vi "PMLambda-Conct Rev A.vi"(0 "Case0:NewFWNone":bool, 1 "Case1:NewFWRed":bool, 2 "Case2:NewFW780":bool, 3 "Case3:NewFW850":bool, 4 "Case4:OldFWRed\nElse5:FW error":bool, 5 "error in":errorcluster, 6 "Supply Cnt":i32=1 min=1 max=5 step=1, 7 "N Systems":i32=1 min=1 max=8 step=1, 8 "COM Ref In":refnum<vi>, 10 "Msg Ref In":refnum<vi>, 11 "Loop Index":i32) -> (14 "Re-conf Lambda?":bool, 15 "Lambda, nm":i32, 19 "error out":errorcluster)   [LabVIEW 2017]
panel:
  # "Inputs"
  # "Outputs"
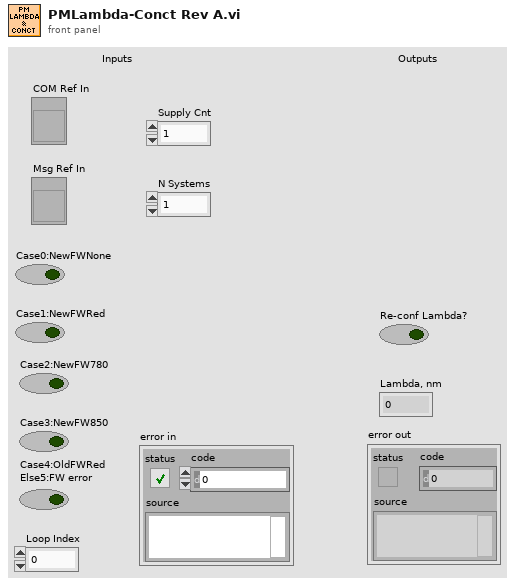
[diagram p1: front panel]
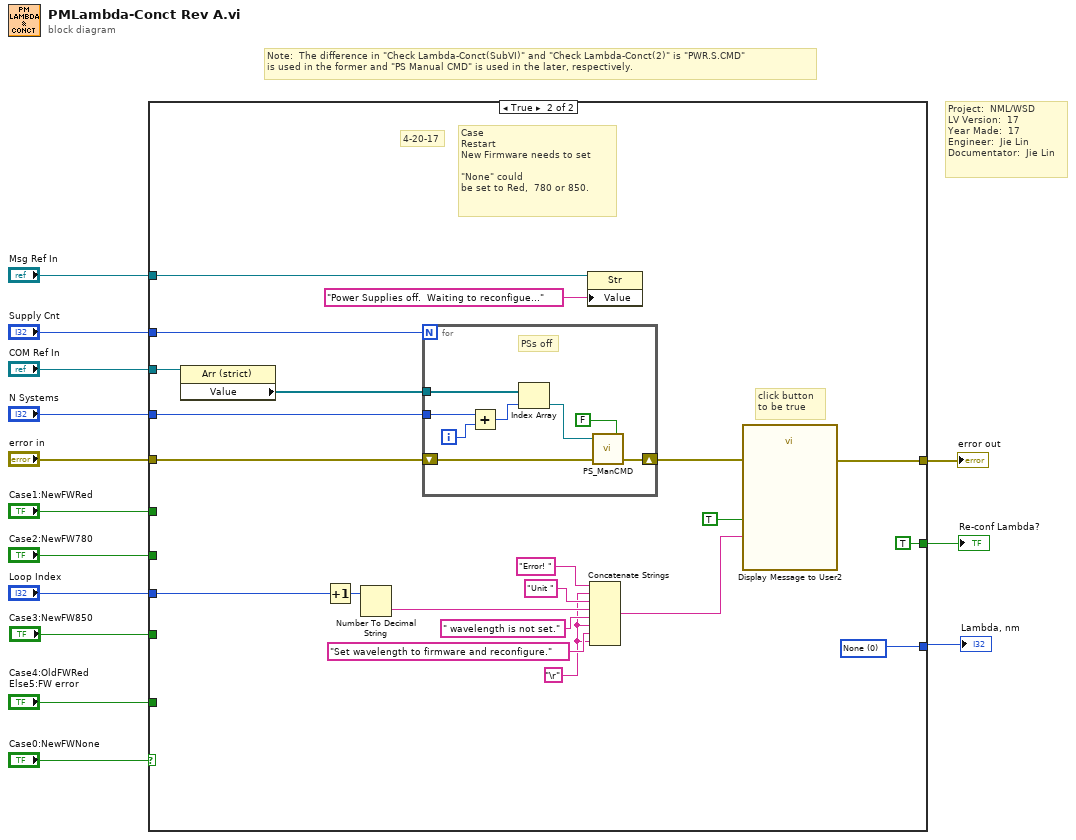
[diagram p0: block diagram]
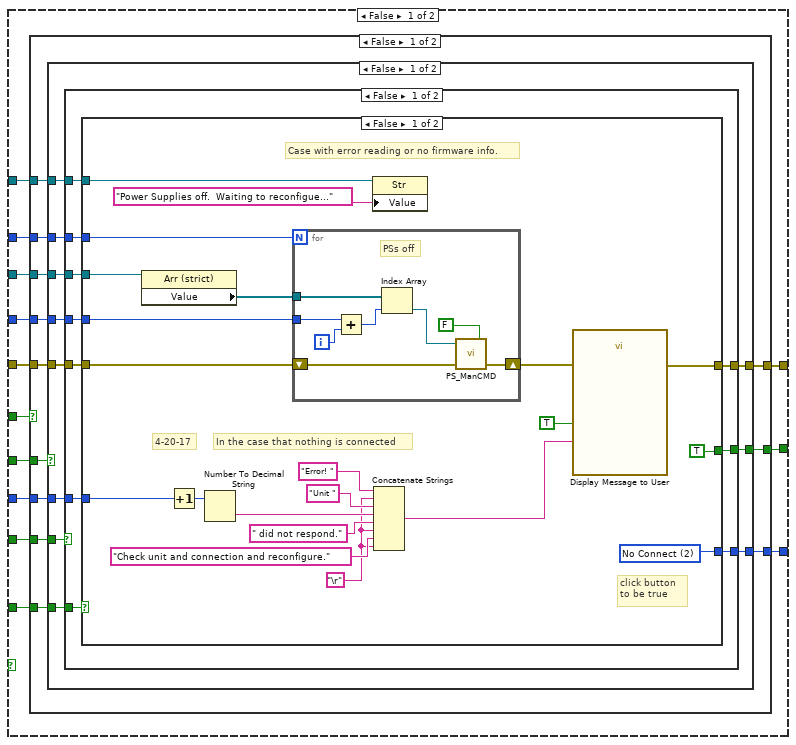
[diagram p2: hidden frame]
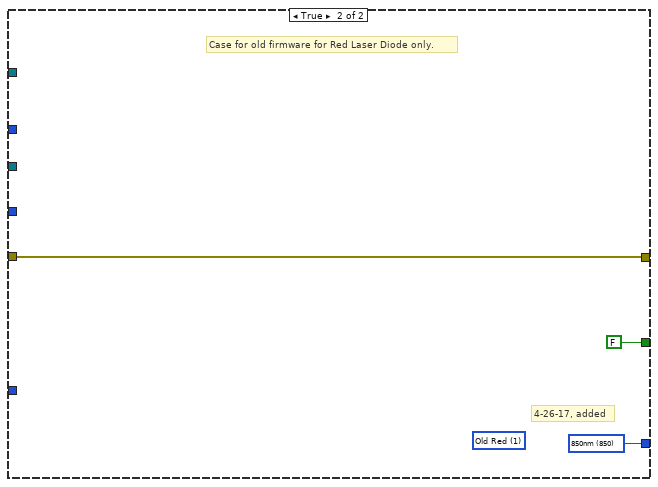
[diagram p3: hidden frame]
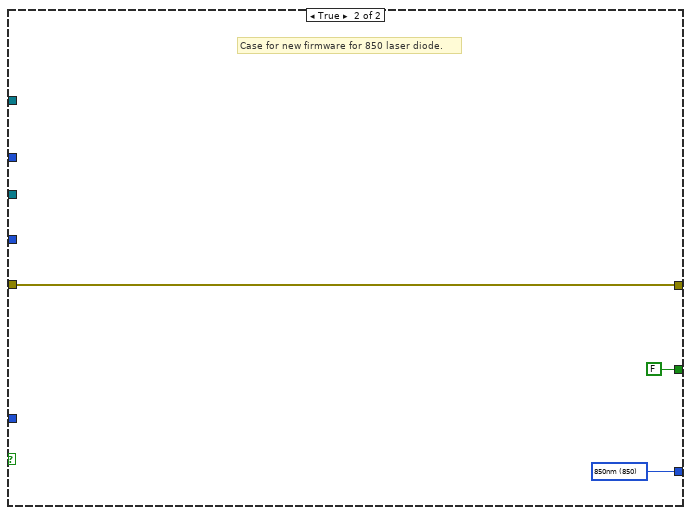
[diagram p4: hidden frame]
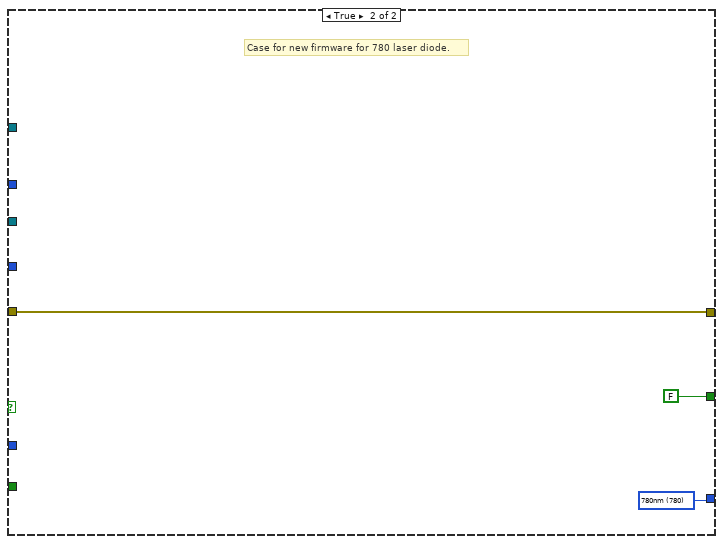
[diagram p5: hidden frame]
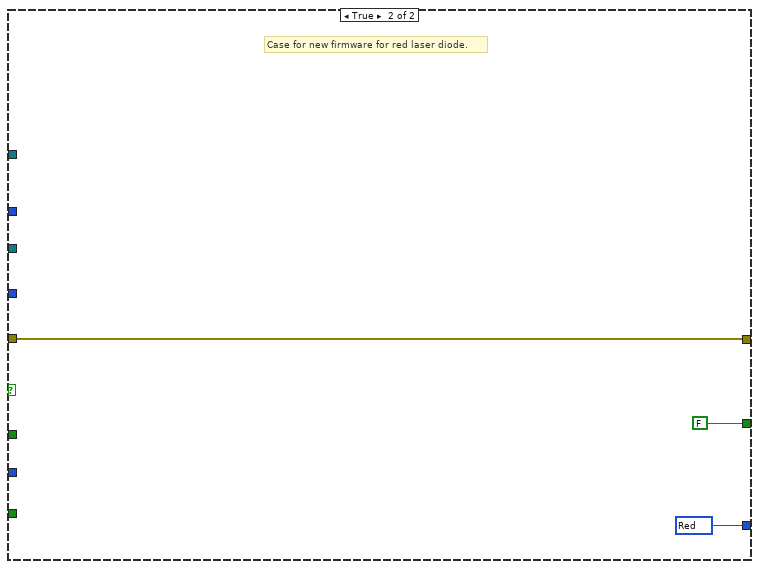
[diagram p6: hidden frame]
diagram:
  # "Project:  NML/WSD \nLV Version:  17\nYear Made:  17\nEngineer:  Jie Lin\nDocumentator:  Jie Lin"
  # "Note:  The difference in \"Check Lambda-Conct(SubVI)\" and \"Check Lambda-Conct(2)\" is \"PWR.S.CMD\" \nis used in the former and \"PS Manual CMD\" is used in the later, respectively."
  n1 = case shown="True" "Case0:NewFWNone" {
    tunnel: [w26 w122] -> w7
    tunnel: "Case1:NewFWRed" -> [w27 _]
    tunnel: "Case2:NewFW780" -> [w25 _]
    tunnel: "Case3:NewFW850" -> [w24 _]
    tunnel: "Case4:OldFWRed\nElse5:FW error" -> [w23 _]
    tunnel: "Loop Index" -> [w17 w113]
    tunnel: [w22 TRUE ("Restart Test")] -> w14
    tunnel: "COM Ref In" -> [w21 w107]
    tunnel: "Msg Ref In" -> [w20 w106]
    tunnel: "error in" -> [w18 w105]
    tunnel: [w19 w104] -> w3
    tunnel: "Supply Cnt" -> [w16 w103]
    tunnel: "N Systems" -> [w15 w102]
    frame False {
      n2 = case shown="False" w27 {
        tunnel: [w38 w100] -> w26
        tunnel: w25 -> [w39 _]
        tunnel: w24 -> [w37 _]
        tunnel: w23 -> [w36 _]
        tunnel: [w35 FALSE] -> w22
        tunnel: w21 -> [w34 _]
        tunnel: w20 -> [w33 _]
        tunnel: [w32 w99] -> w19
        tunnel: w18 -> [w31 w99]
        tunnel: w17 -> [w30 _]
        tunnel: w16 -> [w29 _]
        tunnel: w15 -> [w28 _]
        frame False {
          n3 = case shown="False" w39 {
            tunnel: [w49 w97] -> w38
            tunnel: w37 -> [w50 _]
            tunnel: w36 -> [w48 _]
            tunnel: [w47 FALSE] -> w35
            tunnel: w34 -> [w46 _]
            tunnel: w33 -> [w45 _]
            tunnel: [w44 w96] -> w32
            tunnel: w31 -> [w43 w96]
            tunnel: w30 -> [w42 _]
            tunnel: w29 -> [w41 _]
            tunnel: w28 -> [w40 _]
            frame False {
              n4 = case shown="False" w50 {
                tunnel: [w59 w94] -> w49
                tunnel: w48 -> [w60 _]
                tunnel: [w58 FALSE] -> w47
                tunnel: w46 -> [w57 _]
                tunnel: w45 -> [w56 _]
                tunnel: [w55 w93] -> w44
                tunnel: w43 -> [w54 w93]
                tunnel: w42 -> [w53 _]
                tunnel: w41 -> [w52 _]
                tunnel: w40 -> [w51 _]
                frame False {
                  n5 = case shown="False" w60 {
                    tunnel: [w72 w91] -> w59
                    tunnel: [TRUE FALSE] -> w58
                    tunnel: w57 -> [w69 _]
                    tunnel: w56 -> [w68 _]
                    tunnel: [w67 w90] -> w55
                    tunnel: w54 -> [w66 w90]
                    tunnel: w53 -> [w63 _]
                    tunnel: w52 -> [w62 _]
                    tunnel: w51 -> [w61 _]
                    frame False {
                      w72 = 2 items=["None"=0, "Red"=635, "780nm"=780, "850nm"=850, "Old Red"=1, "No Connect"=2]
                      w70 = "\r"
                      # "Case with error reading or no firmware info."
                      # "click button \nto be true"
                      # "In the case that nothing is connected"
                      # "4-20-17"
                      n6 = property class="Arr (strict)"(reference=w69) -> ("Value"=w64:refnum<visa-resource-name>[])  [unwired: 1 in, 2 out]
                      n7 = Increment(x=w63) -> (x+1=w81:i32)
                      n8 = Number To Decimal String(number=w81) -> (decimal integer string=w77:string)  [unwired: 1 in]
                      n9 = for {
                        N: w62 -> [_]
                        tunnel: w64 -> [w89]
                        shift-right: [w88] -> w65
                        shift-left: w66 -> [w87]
                        tunnel: w61 -> [w82]
                        i -> [w84]
                        # "PSs off"
                        n10 = Add(x=w82, y=w84) -> (x+y=w83:i32)
                        n11 = Index Array(array=w89, index=w83) -> (element=w85:refnum<visa-resource-name>)
                        n12 = call "PS_ManCMD.vi"("Power Sup: T-On/F-Off"=FALSE, "error in"=w87, "VISA resource name"=w85) -> ("error out"=w88:errorcluster)  [unwired: 2 in]
                      }
                      n13 = property class="Str"(reference=w68, "Value"="Power Supplies off.  Waiting to reconfigue..." ("Msg")) -> ()  [unwired: 1 in, 2 out]
                      n14 = Concatenate Strings("Error! " ("string"), w70, "Unit " ("string"), w77, " did not respond." ("string"), w70, "Check unit and connection and reconfigure." ("string"), w70) -> (w78:string)
                      n15 = call "Display Message to User"("error in (no error)"=w65, "Enable"=TRUE, "Message"=w78) -> ("error out"=w67:errorcluster)  [unwired: 7 in, 1 out]
                    }
                    frame True {
                      (unwired) 1 items=["None"=0, "Red"=635, "780nm"=780, "850nm"=850, "Old Red"=1, "No Connect"=2]
                      w91 = 850 items=["None"=0, "Red"=635, "780nm"=780, "850nm"=850, "Old Red"=1, "No Connect"=2]
                      # "Case for old firmware for Red Laser Diode only."
                      # "4-26-17, added"
                    }
                  }
                }
                frame True {
                  w94 = 850 items=["None"=0, "Red"=635, "780nm"=780, "850nm"=850, "Old Red"=1, "No Connect"=2]
                  # "Case for new firmware for 850 laser diode."
                }
              }
            }
            frame True {
              w97 = 780 items=["None"=0, "Red"=635, "780nm"=780, "850nm"=850, "Old Red"=1, "No Connect"=2]
              # "Case for new firmware for 780 laser diode."
            }
          }
        }
        frame True {
          w100 = 635 items=["None"=0, "Red"=635, "780nm"=780, "850nm"=850, "Old Red"=1, "No Connect"=2]
          # "Case for new firmware for red laser diode."
        }
      }
    }
    frame True {
      w108 = "\r"
      w122 = 0 items=["None"=0, "Red"=635, "780nm"=780, "850nm"=850, "Old Red"=1, "No Connect"=2]
      # "click button \nto be true"
      # "4-20-17"
      # "Case \nRestart\nNew Firmware needs to set\n\n\"None\" could\nbe set to Red,  780 or 850."
      n16 = property class="Arr (strict)"(reference=w107) -> ("Value"=w112:refnum<visa-resource-name>[])  [unwired: 1 in, 2 out]
      n17 = Increment(x=w113) -> (x+1=w121:i32)
      n18 = Number To Decimal String(number=w121) -> (decimal integer string=w117:string)  [unwired: 1 in]
      n19 = for {
        N: w103 -> [_]
        tunnel: w112 -> [w130]
        shift-right: [w129] -> w111
        shift-left: w105 -> [w128]
        tunnel: w102 -> [w123]
        i -> [w125]
        # "PSs off"
        n20 = Add(x=w123, y=w125) -> (x+y=w124:i32)
        n21 = Index Array(array=w130, index=w124) -> (element=w126:refnum<visa-resource-name>)
        n22 = call "PS_ManCMD.vi"("Power Sup: T-On/F-Off"=FALSE, "error in"=w128, "VISA resource name"=w126) -> ("error out"=w129:errorcluster)  [unwired: 2 in]
      }
      n23 = property class="Str"(reference=w106, "Value"="Power Supplies off.  Waiting to reconfigue..." ("Msg")) -> ()  [unwired: 1 in, 2 out]
      n24 = Concatenate Strings("Error! " ("string"), w108, "Unit " ("string"), w117, " wavelength is not set." ("string"), w108, "Set wavelength to firmware and reconfigure." ("string"), w108) -> (w118:string)
      n25 = call "Display Message to User2"("error in (no error)"=w111, "Enable"=TRUE, "Message"=w118) -> ("error out"=w104:errorcluster)  [unwired: 7 in, 1 out]
    }
  }
  "Re-conf Lambda?" <- w14
  "Lambda, nm" <- w7
  "error out" <- w3
